vi "Measure Output.vi"(8 "error in":errorcluster, 11 "57XX in":refnum<class "57XX.lvclass">) -> (0 "error out":errorcluster, 1 "Current":dbl[](array[numeric]), 2 "Voltage":dbl[](array[numeric]), 3 "57XX out":refnum<class "57XX.lvclass">)   [LabVIEW 2019, in "57XX.lvlib" / "57XX.lvclass"]
doc: "Child classes must override this VI:\n\nThis VI is the device specific query of current and voltage measurements. \nThe return values are: \nVoltage Array - One voltage measurement per channel single channel supplies should only return a single array element\nCurrent Array - - One current measurement per channel single channel supplies should only return a single array element"
uses:
  Library/57XX.lvclass
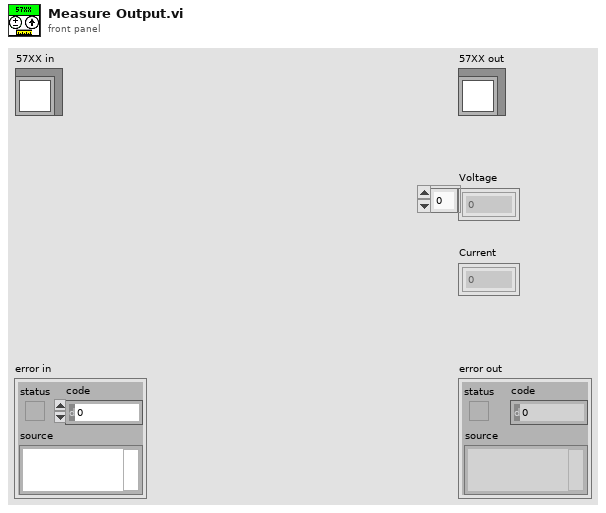
[diagram p1: front panel]
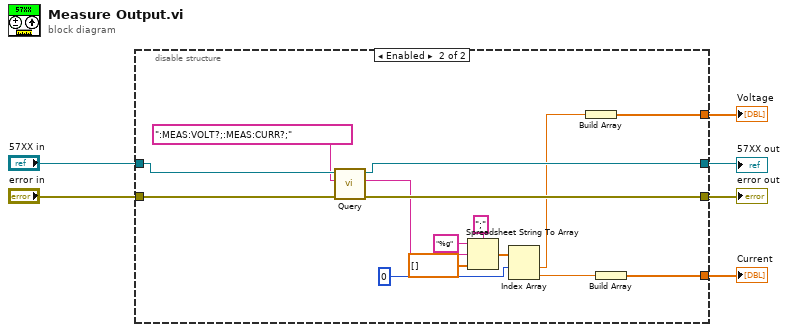
[diagram p0: block diagram]
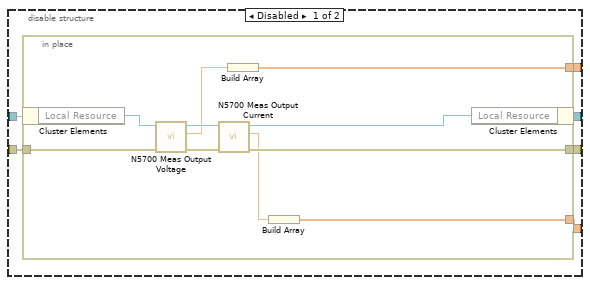
[diagram p2: hidden frame]
diagram:
  n1 = disable-structure shown="Enabled" {
    disable-tunnel: "57XX in" -> [w12 w36]
    disable-tunnel: [w11 w33] -> w5
    disable-tunnel: [w10 w34] -> w4
    disable-tunnel: "error in" -> [w9 w37]
    disable-tunnel: [w8 w24] -> w2
    disable-tunnel: [w7 w25] -> w1
    frame Disabled {
      n2 = in-place {
        in-place-border: [w18] -> w11
        in-place-border: w9 -> [w17]
        in-place-border: [w14] -> w8
        in-place-border: [w13] -> w7
        n3 = in-place-cluster #1(w12) -> ("Local Resource"=w20:refnum<visa-resource-name>)
        n4 = call <instrlib>:"N5700 Meas Output Voltage.vi"("error"=w17, "VISA"=w20) -> ("error out"=w22:errorcluster, "Output Voltage"=w16:dbl, "VISA out"=w21:refnum<visa-resource-name>)  [unwired: 4 in]
        n5 = call <instrlib>:"N5700 Meas Output Current.vi"("error"=w22, "VISA"=w21) -> ("error out"=w18:errorcluster, "Output Current"=w15:dbl, "VISA out"=w19:refnum<visa-resource-name>)  [unwired: 4 in]
        n6 = Build Array(w16) -> (w13:dbl[])
        n7 = Build Array(w15) -> (w14:dbl[])
        n8 = in-place-cluster #1("Local Resource"=w19) -> (w10:refnum<class "57XX.lvclass">)
      }
    }
    frame Enabled {
      n9 = call "Query.vi"("error in"=w37, "Write in"=":MEAS:VOLT?;:MEAS:CURR?;", "57XX in"=w36) -> ("error out"=w33:errorcluster, "Read out"=w23:string, "57XX out"=w34:refnum<class "57XX.lvclass">)  [unwired: 6 in]
      n10 = Spreadsheet String To Array(delimiter (Tab)=";", format string="%g", spreadsheet string=w23, array type (2D Dbl)=dbl[] []) -> (array=w31:dbl[])
      n11 = Index Array(array=w31, index #1=0 ("index")) -> (element #1=w29:dbl, element #2=w28:dbl)  [unwired: 1 in]
      n12 = Build Array(w29) -> (w25:dbl[])
      n13 = Build Array(w28) -> (w24:dbl[])
    }
  }
  "error out" <- w5
  "57XX out" <- w4
  "Current" <- w2
  "Voltage" <- w1
